vi "Send Receive New Subscription.vi"(7 "Message Priority (Normal)":T1=enum."Normal", 8 "error in (no error)":errorcluster, 9 "Topic":string, 10 "Name":string, 11 "Message Enqueuer":refnum<class "Message Enqueuer.lvclass">) -> (0 "error out":errorcluster, 3 "Message Enqueuer out":refnum<class "Message Enqueuer.lvclass">)   [LabVIEW 2020, in "Actor Pub Sub Channels.lvlib" / "Receive New Subscription Msg.lvclass"]
doc: "This VI sends the message to an actor."
uses:
  Receive New Subscription Msg.lvclass
  <vilib>/ActorFramework/Message Enqueuer/Message Enqueuer.lvclass
  <vilib>/ActorFramework/Message Enqueuer/Message Priority.ctl
  C:/Program Files (x86)/National Instruments/LabVIEW 2020/vi.lib/ActorFramework/Message/Message.lvclass
  Receive New Subscription Msg.lvclass/Receive New Subscription Msg.ctl
  <vilib>/ActorFramework/Message Enqueuer/Message Enqueuer.lvclass/Message Enqueuer.ctl
  <vilib>/ActorFramework/Message Priority Queue/Priority Enqueue.vi
  C:/Users/Simon/Documents/GitHub/LV-Actor-Pub-Sub/Source/Actor Pub Sub Channels/PubSub Status Reciever Interface Messages/Recieve New Subscription Msg/Receive New Subscription Msg.lvclass
  C:/Users/Simon/Documents/GitHub/LV-Actor-Pub-Sub/Source/Actor Pub Sub Channels/Pub Sub Status Message/Pub Sub Status Message.lvclass
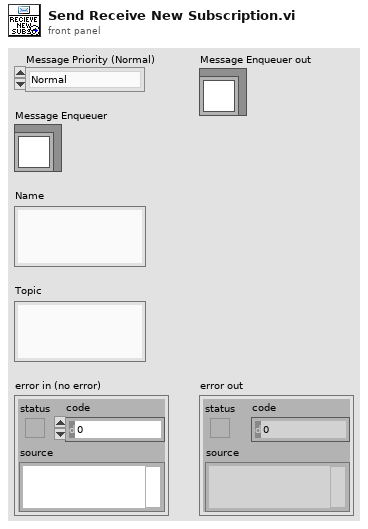
[diagram p1: front panel]
types:
  T1 = typedef "Actor Framework.lvlib/Message Enqueuer.lvclass/Message Priority.ctl" = enum16{"Low", "Normal", "High"}
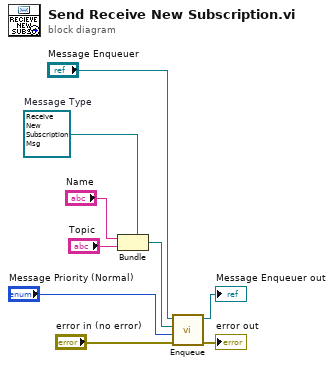
[diagram p0: block diagram]
diagram:
  w6 = refnum<class "Receive New Subscription Msg.lvclass"> refnum  # Message Type
  n1 = Bundle(cluster=w6, "Name", "Topic") -> (w5:refnum<class "Receive New Subscription Msg.lvclass">)
  n2 = call <vilib>:"Enqueue.vi"("error in (no error)"="error in (no error)", "Message Priority (Normal)"="Message Priority (Normal)", "Message"=w5, "Message Enqueuer in"="Message Enqueuer") -> ("error out"=→"error out":errorcluster, "Message Enqueuer out"=→"Message Enqueuer out":refnum<class "Message Enqueuer.lvclass">)  [unwired: 6 in]
